vi "KGN Get Info.vi"(8 "Fehler (Eingang, kein Fehler)":errorcluster, 10 "VISA-Ressourcenname":refnum<visa-resource-name>, 11 "device":u32) -> (0 "Fehler (Ausgang)":errorcluster, 1 "System Cluster":T1, 2 "VISA-Ressourcenname out":refnum<visa-resource-name>, 3 "dup device":u32, 4 "Kommandos gesendet":string)   [LabVIEW 2020, in "Linearisierung v2.lvlib" / "Gasteiler.lvlib" / "HovaCAL_Interface.lvlib" / "KGN.lvlib" / "KGN GUI Get.lvlib"]
uses:
  KGN GUI Get.lvlib
  Controls/Info Cluster.ctl
  get/get.lvlib
  Controls/Controls.lvlib
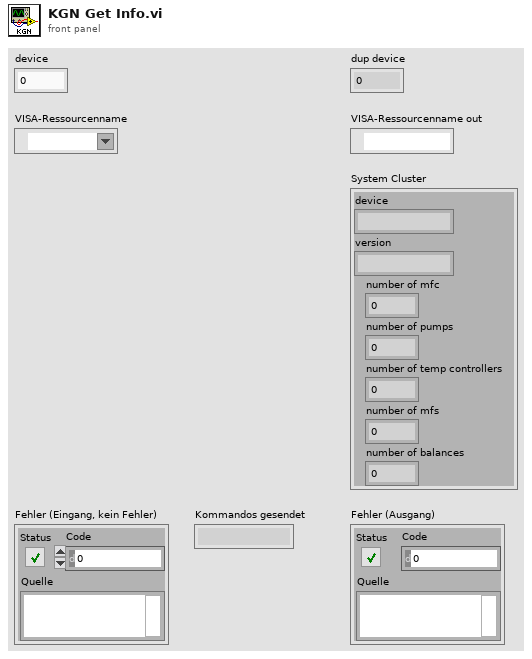
[diagram p1: front panel]
types:
  T1 = typedef "Linearisierung v2.lvlib/Gasteiler.lvlib/HovaCAL_Interface.lvlib/Controls.lvlib/Info Cluster.ctl" = cluster{"device":string, "version":string, "number of mfc":i32, "number of pumps":i32, "number of temp controllers":i32, "number of mfs":i32, "number of balances":i32}
  T2 = cluster{"device":string, "version":string, "number of mfc":i32, "number of pumps":i32, "number of temp controllers":i32, "number of mfs":i32, "number of balances":i32}
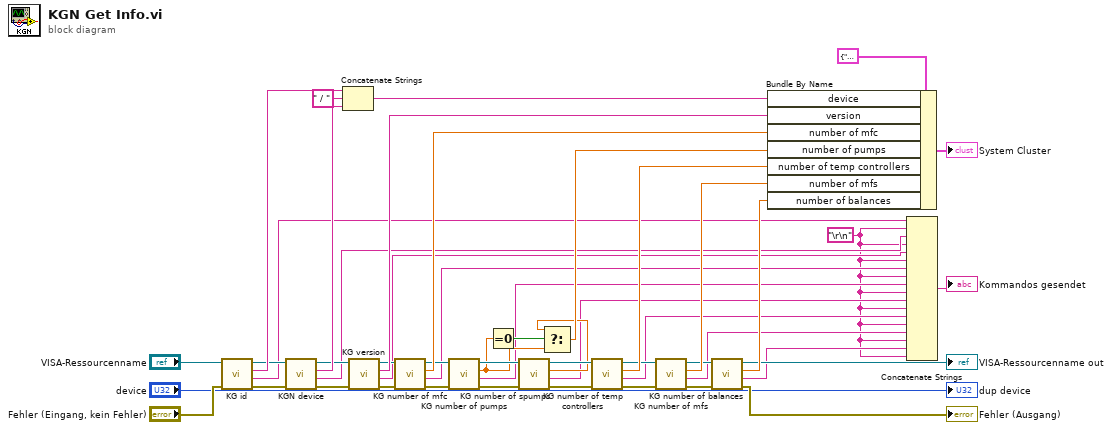
[diagram p0: block diagram]
diagram:
  w1 = "\r\n"
  n1 = call "KG id.vi"("Fehler (Eingang, kein Fehler)"="Fehler (Eingang, kein Fehler)", "VISA-Ressourcenname"="VISA-Ressourcenname") -> ("Fehler (Ausgang)"=w29:errorcluster, "Kommando gesendet"=w11:string, "Id"=w34:string, "VISA-Ressourcenname (Ausgang)"=w30:refnum<visa-resource-name>)  [unwired: 6 in]
  n2 = call "KGN device.vi"("Fehler (Eingang, kein Fehler)"=w29, "VISA-Ressourcenname"=w30) -> ("Fehler (Ausgang)"=w27:errorcluster, "Kommando gesendet"=w10:string, "Device"=w46:string, "VISA-Ressourcenname (Ausgang)"=w28:refnum<visa-resource-name>)  [unwired: 6 in]
  n3 = Concatenate Strings(w34, " / " ("String"), w46) -> (w35:string)
  n4 = call "KG version.vi"("Fehler (Eingang, kein Fehler)"=w27, "VISA-Ressourcenname"=w28) -> ("Fehler (Ausgang)"=w25:errorcluster, "Kommando gesendet"=w9:string, "Version"=w47:string, "VISA-Ressourcenname (Ausgang)"=w26:refnum<visa-resource-name>)  [unwired: 6 in]
  n5 = call "KG number of mfc.vi"("Fehler (Eingang, kein Fehler)"=w25, "VISA-Ressourcenname"=w26) -> ("Fehler (Ausgang)"=w18:errorcluster, "Kommando gesendet"=w8:string, "number of mfc"=w43:dbl, "VISA-Ressourcenname (Ausgang)"=w24:refnum<visa-resource-name>)  [unwired: 6 in]
  n6 = call "KG number of pumps.vi"("Fehler (Eingang, kein Fehler)"=w18, "VISA-Ressourcenname"=w24) -> ("Fehler (Ausgang)"=w19:errorcluster, "Kommando gesendet"=w7:string, "number of pumps"=w13:dbl, "VISA-Ressourcenname (Ausgang)"=w23:refnum<visa-resource-name>)  [unwired: 6 in]
  n7 = Equal To 0?(x=w13) -> (x = 0?=w14:bool)
  n8 = call "KG number of spumps.vi"("Fehler (Eingang, kein Fehler)"=w19, "VISA-Ressourcenname"=w23) -> ("Fehler (Ausgang)"=w17:errorcluster, "Kommando gesendet"=w6:string, "number of spumps"=w12:dbl, "VISA-Ressourcenname (Ausgang)"=w22:refnum<visa-resource-name>)  [unwired: 6 in]
  n9 = Select(t=w12, s=w14, f=w13) -> (s? t:f=w42:dbl)
  n10 = call "KG number of temp controllers.vi"("Fehler (Eingang, kein Fehler)"=w17, "VISA-Ressourcenname"=w22) -> ("Fehler (Ausgang)"=w16:errorcluster, "Kommando gesendet"=w5:string, "number of temp controllers"=w41:dbl, "VISA-Ressourcenname (Ausgang)"=w21:refnum<visa-resource-name>)  [unwired: 6 in]
  n11 = call "KG number of mfs.vi"("Fehler (Eingang, kein Fehler)"=w16, "VISA-Ressourcenname"=w21) -> ("Fehler (Ausgang)"=w15:errorcluster, "Kommando gesendet"=w4:string, "number of mfs"=w40:dbl, "VISA-Ressourcenname (Ausgang)"=w20:refnum<visa-resource-name>)  [unwired: 6 in]
  n12 = call "KG number of balances.vi"("Fehler (Eingang, kein Fehler)"=w15, "VISA-Ressourcenname"=w20) -> ("Fehler (Ausgang)"=→"Fehler (Ausgang)":errorcluster, "Kommando gesendet"=w3:string, "number of balances"=w39:dbl, "VISA-Ressourcenname (Ausgang)"=→"VISA-Ressourcenname out":refnum<visa-resource-name>)  [unwired: 6 in]
  n13 = Bundle By Name(cluster=T2 {"device"="", "version"="", "number of mfc"=0, "number of pumps"=0, "number of temp controllers"=0, "number of mfs"=0, "number of balances"=0} ("Info Cluster"), "device"=w35, "version"=w47, "number of mfc"=w43, "number of pumps"=w42, "number of temp controllers"=w41, "number of mfs"=w40, "number of balances"=w39) -> (→"System Cluster":T2)
  n14 = Concatenate Strings(w11, w1, w10, w1, w9, w1, w8, w1, w7, w1, w6, w1, w5, w1, w4, w1, w3, w1) -> (→"Kommandos gesendet":string)
  "dup device" <- "device"
